vi "Bundle by name.vi"(10 "Property Reference":refnum<vi>[](array[refnum]), 11 "Cluster Constant reference":refnum<vi>) -> ()   [LabVIEW 2015]
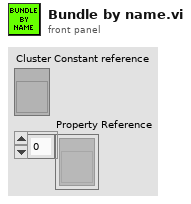
[diagram p1: front panel]
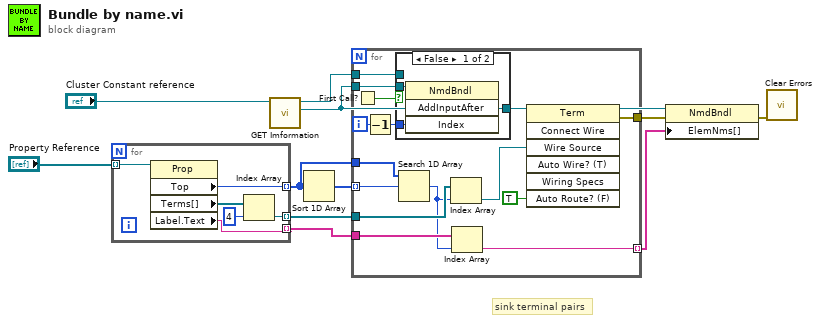
[diagram p0: block diagram]
diagram:
  # "sink terminal pairs"
  n1 = for {
    tunnel: "Property Reference" -> [w15] mode=indexing
    tunnel: [w14] -> w4 mode=indexing
    tunnel: [w13] -> w5 mode=indexing
    tunnel: [w12] -> w3 mode=indexing
    n2 = property class="Prop"(reference=w15) -> ("Top"=w13:i32, "Terms[]"=w17:refnum<vi>[], "Label.Text"=w12:string)  [unwired: 1 in, 2 out]
    n3 = Index Array(array=w17, index=4) -> (element=w14:refnum<vi>)
  }
  n4 = call "GET Imformation.vi"("Cluster Constant reference"="Cluster Constant reference") -> ("Bundle Reference"=w2:refnum<vi>, "Term Refnum"=w1:refnum<vi>)  [unwired: 9 in]
  n5 = Sort 1D Array(array=w5) -> (sorted array=w11:i32[])
  n6 = for {
    tunnel: w11 -> [w30] mode=indexing
    tunnel: w4 -> [w32]
    tunnel: w5 -> [w31]
    tunnel: w1 -> [w27]
    tunnel: w2 -> [w26]
    tunnel: [w19] -> w10 mode=indexing
    tunnel: [w22] -> w9
    tunnel: w3 -> [w21]
    i -> [w25]
    n7 = First Call?() -> (First Call?: T/F=w29:bool)
    n8 = Decrement(x=w25) -> (x-1=w28:i32)
    n9 = case shown="False" w29 {
      tunnel: w26 -> [w35 _]
      tunnel: w28 -> [w34 _]
      tunnel: [w33 w36] -> w24
      tunnel: w27 -> [_ w36]
      frame False {
        n10 = invoke class="NmdBndl" method="AddInputAfter"(reference=w35, "Index"=w34) -> ("AddInputAfter"=w33:refnum<vi>)  [unwired: 2 in, 3 out]
      }
      frame True {
      }
    }
    n11 = Search 1D Array(1D array=w31, element=w30) -> (index of element=w20:i32)  [unwired: 1 in]
    n12 = Index Array(array=w32, index=w20) -> (element=w23:refnum<vi>)
    n13 = Index Array(array=w21, index=w20) -> (element=w19:string)
    n14 = invoke class="Term" method="Connect Wire"(reference=w24, "Wire Source"=w23, "Auto Route? (F)"=TRUE) -> (error out=w22:errorcluster)  [unwired: 4 in, 6 out]
  }
  n15 = property class="NmdBndl"(reference=w2, error in=w9, "ElemNms[]"=w10) -> (error out=w8:errorcluster)  [unwired: 1 out]
  n16 = call <vilib>:"Clear Errors.vi"("error in (no error)"=w8) -> ()  [unwired: 5 in, 2 out]
